vi "DAC Save Results.vi"(8 "error in":errorcluster, 9 "Log Details?":bool, 10 "tdms file":refnum<k34>, 11 "DAC Heater Ctrl in":refnum<class "DAC Heater Ctrl.lvclass">) -> (0 "error out":errorcluster)   [LabVIEW 2019, in "DAC.lvlib" / "DAC Heater Ctrl.lvclass"]
uses:
  DAC Heater Ctrl.lvclass
  C:/Users/wg/Documents/LV_Projects/TestStand/App/DAC/DAC.lvclass
  DAC.lvclass/DAC.ctl
  DAC Heater Ctrl.lvclass/DAC Heater Ctrl.ctl
  DAC.lvclass
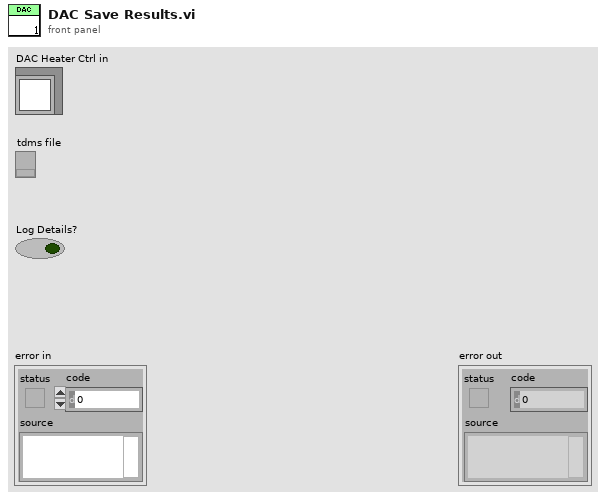
[diagram p1: front panel]
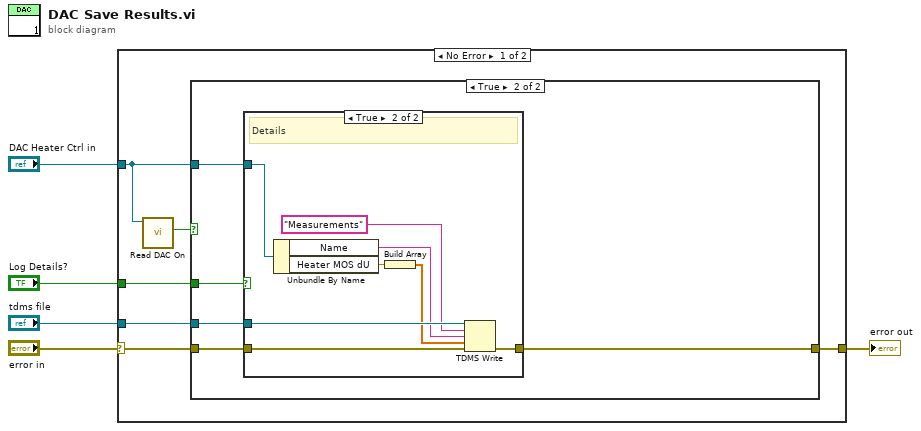
[diagram p0: block diagram]
diagram:
  n1 = case shown="No Error" "error in" {
    selector: "error in" -> [w8 w27]
    tunnel: "DAC Heater Ctrl in" -> [w11 _]
    tunnel: "tdms file" -> [w9 _]
    tunnel: [w7 w27] -> w3
    tunnel: "Log Details?" -> [w6 _]
    frame No Error {
      n2 = call "Read DAC On.vi"("DAC in"=w11) -> ("DAC On"=w10:bool)  [unwired: 8 in, 2 out]
      n3 = case shown="True" w10 {
        tunnel: w11 -> [_ w16]
        tunnel: w9 -> [_ w14]
        tunnel: w8 -> [w12 w15]
        tunnel: [w12 w17] -> w7
        tunnel: w6 -> [_ w13]
        frame False {
        }
        frame True {
          n4 = case shown="True" w13 {
            tunnel: w14 -> [_ w26]
            tunnel: w15 -> [w18 w21]
            tunnel: w16 -> [_ w19]
            tunnel: [w18 w20] -> w17
            frame False {
            }
            frame True {
              # "Details"
              n5 = Unbundle By Name(w19) -> ("Name"=w23:string, "Heater MOS dU"=w25:dbl)
              n6 = Build Array(w25) -> (w24:dbl[])
              n7 = TDMS Write(0:w26, 5:"Measurements" ("group name in (Untitled)"), 7:w23, 9:w24, 11:w21) -> (15:w20:errorcluster)  [unwired: 1 in, 3 out]
            }
          }
        }
      }
    }
    frame Error {
    }
  }
  "error out" <- w3
